vi "Serial Verify.vi"(6 "Function Choose":T3(ring), 8 "error in (no error)":errorcluster, 9 "Config Parameters":T1={"HEX_Max"="1A", "HEX_Min"="", "Read?"=FALSE, "write buffer"="", "Wait Time(ms)"=0}, 10 "Serial Config":T2={"baud rate (9600)"=9600, "stop bits (10: 1 bit)"=10, "flow control (0:none)"=0, "data bits (8)"=8, "parity (0:none)"=enum."None"} {"data bits (8)" min=5 max=8 step=1; "flow control (0:none)" items=["None", "XON/XOFF", "RTS/CTS", "XON/XOFF & RTS/CTS", "DTR/DSR", "XON/XOFF & DTR/DSR"]; "stop bits (10: 1 bit)" items=["1.0"=10, "1.5"=15, "2.0"=20]}, 11 "VISA resource name":refnum<visa-resource-name>) -> (0 "error out":errorcluster, 2 "Result":string, 3 "VISA resource name out":refnum<visa-resource-name>)   [LabVIEW 2020]
uses:
  6da304eb-4ed6-4a05-99e3-1c15b644af6c.vi
  a31ce7cd-64d5-4b98-9705-88e585e787fb.vi
  <vilib>/Instr/_visa.llb/VISA Configure Serial Port (Instr).vi
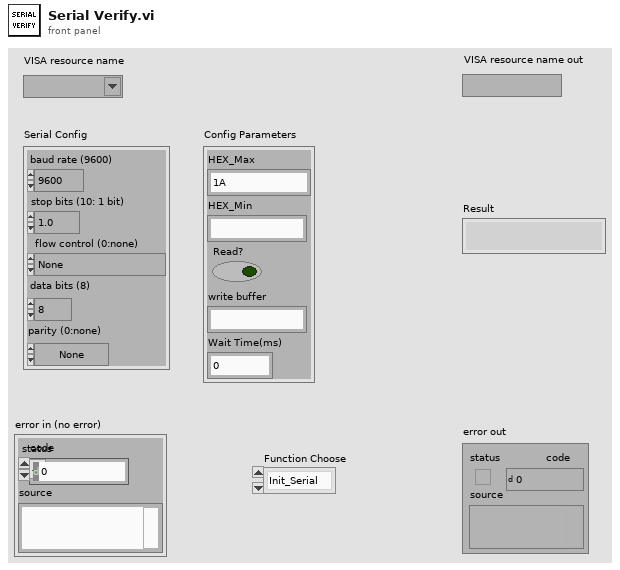
[diagram p1: front panel]
types:
  T1 = cluster{"HEX_Max":string, "HEX_Min":string, "Read?":bool, "write buffer":string, "Wait Time(ms)":u32}
  T2 = cluster{"baud rate (9600)":u32, "stop bits (10: 1 bit)":u16, "flow control (0:none)":u16, "data bits (8)":u16, "parity (0:none)":enum16{"None", "Odd", "Even", "Mark", "Space"}}
  T3 = enum16{"Init_Serial", "Write&Read", "Check_Value", "Close_Serial"}
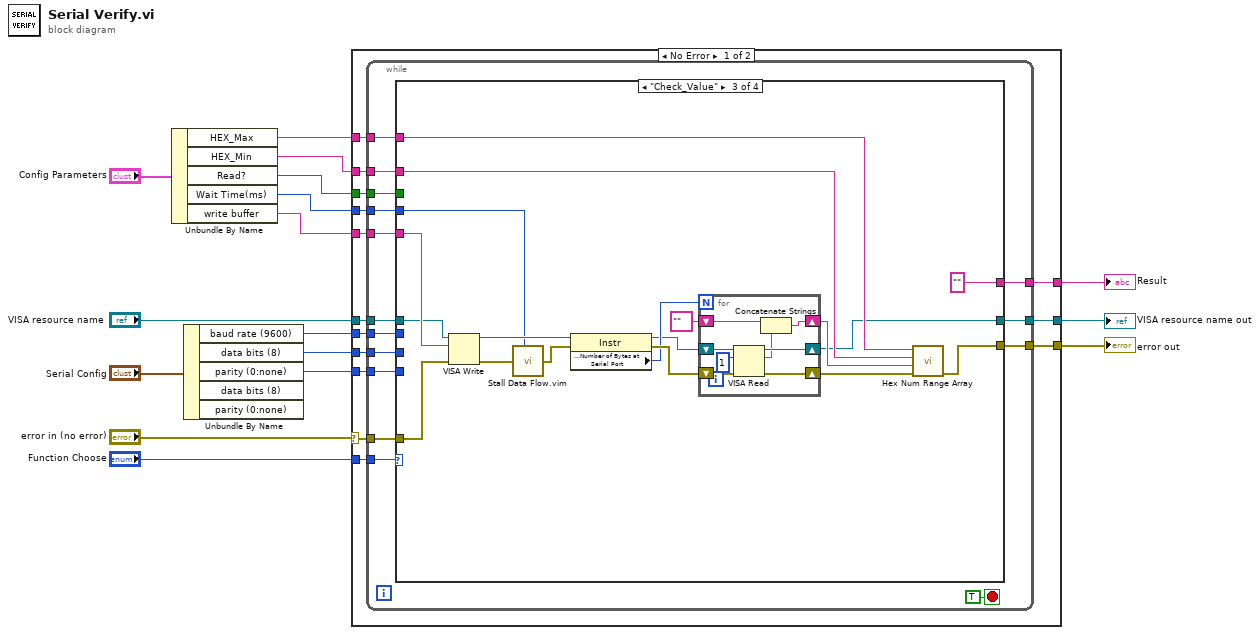
[diagram p0: block diagram]
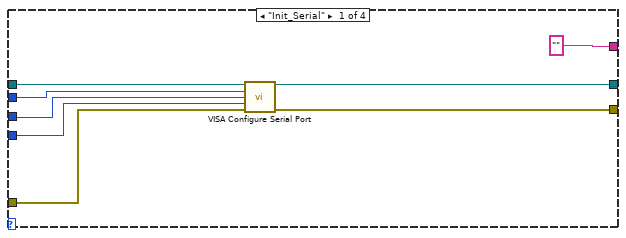
[diagram p2: hidden frame]
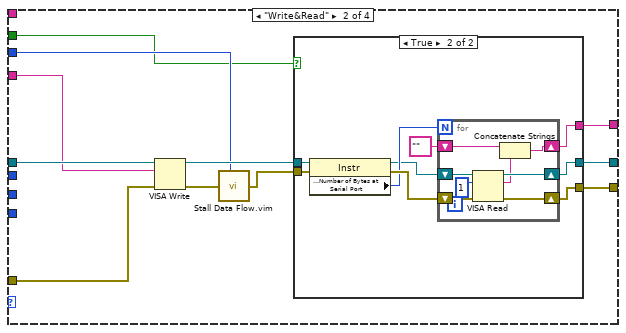
[diagram p3: hidden frame]
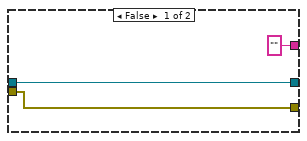
[diagram p4: hidden frame]
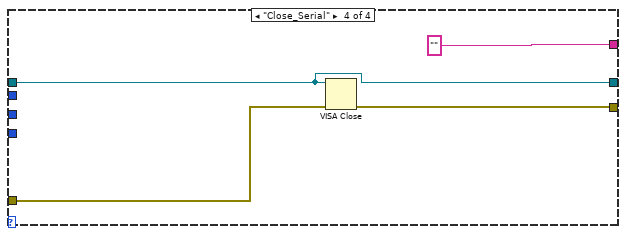
[diagram p5: hidden frame]
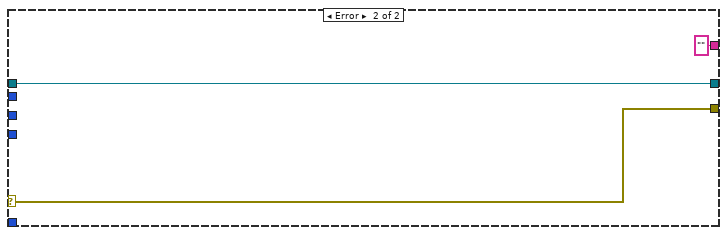
[diagram p6: hidden frame]
diagram:
  n1 = Unbundle By Name("Config Parameters") -> ("HEX_Max"=w5:string, "HEX_Min"=w4:string, "Read?"=w3:bool, "Wait Time(ms)"=w2:u32, "write buffer"=w1:string)
  n2 = Unbundle By Name("Serial Config") -> ("baud rate (9600)"=w12:u32, "data bits (8)"=w11:u16, "parity (0:none)"=w10:enum16{"None", "Odd", "Even", "Mark", "Space"})  [unwired: 2 out]
  n3 = case shown="No Error" "error in (no error)" {
    selector: "error in (no error)" -> [w25 w115]
    tunnel: "Function Choose" -> [w30 _]
    tunnel: "VISA resource name" -> [w29 w116]
    tunnel: w12 -> [w28 _]
    tunnel: w11 -> [w27 _]
    tunnel: w10 -> [w26 _]
    tunnel: [w24 w115] -> w9
    tunnel: [w23 w116] -> w8
    tunnel: w2 -> [w22 _]
    tunnel: w1 -> [w21 _]
    tunnel: [w20 ""] -> w7
    tunnel: w3 -> [w19 _]
    tunnel: w5 -> [w18 _]
    tunnel: w4 -> [w17 _]
    frame No Error {
      n4 = while {
        tunnel: w30 -> [w37]
        tunnel: w29 -> [w44]
        tunnel: w28 -> [w43]
        tunnel: w27 -> [w42]
        tunnel: w26 -> [w41]
        tunnel: w25 -> [w40]
        tunnel: [w39] -> w24
        tunnel: [w38] -> w23
        tunnel: w22 -> [w36]
        tunnel: w21 -> [w35]
        tunnel: [w34] -> w20
        tunnel: w19 -> [w33]
        tunnel: w18 -> [w32]
        tunnel: w17 -> [w31]
        stop <- TRUE stop-if-true
        n5 = case shown="\"Check_Value\"" w37 {
          tunnel: w44 -> [w53 w64 w93 w112]
          tunnel: w43 -> [w52 _ _ _]
          tunnel: w42 -> [w51 _ _ _]
          tunnel: w41 -> [w50 _ _ _]
          tunnel: w40 -> [w49 w63 w95 w114]
          tunnel: [w48 w54 w87 w113] -> w39
          tunnel: [w47 w55 w86 w112] -> w38
          tunnel: w36 -> [_ w59 w92 _]
          tunnel: w35 -> [_ w58 w94 _]
          tunnel: ["" w57 "" ""] -> w34
          tunnel: w33 -> [_ w56 _ _]
          tunnel: w32 -> [_ _ w90 _]
          tunnel: w31 -> [_ _ w89 _]
          frame "Init_Serial" {
            n6 = call-poly "VISA Configure Serial Port"("VISA resource name"=w53, "baud rate (9600)"=w52, "data bits (8)"=w51, "parity (0:none)"=w50, "error in (no error)"=w49) -> ("VISA resource name out"=w47:refnum<visa-resource-name>, "error out"=w48:errorcluster)  [unwired: 9 in]
          }
          frame "Write&Read" {
            n7 = VISA Write(VISA resource name=w64, write buffer=w58, error in (no error)=w63) -> (VISA resource name out=w60:refnum<visa-resource-name>, error out=w62:errorcluster)  [unwired: 1 out]
            n8 = call "Stall Data Flow.vim"("value in"=w62, "milliseconds to wait"=w59) -> ("value out"=w61:errorcluster)  [unwired: 1 out]
            n9 = case shown="True" w56 {
              tunnel: w61 -> [w66 w72]
              tunnel: w60 -> [w67 w71]
              tunnel: ["" w70] -> w57
              tunnel: [w67 w69] -> w55
              tunnel: [w66 w68] -> w54
              frame False {
              }
              frame True {
                n10 = property class="Instr"(reference=w71, error in=w72) -> (reference out=w74:refnum<visa-resource-name>, error out=w76:errorcluster, "Serial Settings:Number of Bytes at Serial Port"=w75:u32)
                n11 = for {
                  N: w75 -> [_]
                  shift-right: [w80] -> w69
                  shift-left: w74 -> [w82]
                  shift-right: [w77] -> w70
                  shift-left: "" -> [w78]
                  shift-right: [w81] -> w68
                  shift-left: w76 -> [w83]
                  n12 = VISA Read(VISA resource name=w82, byte count=u32 1, error in (no error)=w83) -> (VISA resource name out=w80:refnum<visa-resource-name>, read buffer=w79:string, error out=w81:errorcluster)  [unwired: 1 out]
                  n13 = Concatenate Strings(w78, w79) -> (w77:string)
                }
              }
            }
          }
          frame "Check_Value" {
            n14 = VISA Write(VISA resource name=w93, write buffer=w94, error in (no error)=w95) -> (VISA resource name out=w100:refnum<visa-resource-name>, error out=w102:errorcluster)  [unwired: 1 out]
            n15 = call "Stall Data Flow.vim"("value in"=w102, "milliseconds to wait"=w92) -> ("value out"=w101:errorcluster)  [unwired: 1 out]
            n16 = property class="Instr"(reference=w100, error in=w101) -> (reference out=w97:refnum<visa-resource-name>, error out=w99:errorcluster, "Serial Settings:Number of Bytes at Serial Port"=w98:u32)
            n17 = for {
              N: w98 -> [_]
              shift-right: [w106] -> w86
              shift-left: w97 -> [w108]
              shift-right: [w103] -> w88
              shift-left: "" -> [w104]
              shift-right: [w107] -> w91
              shift-left: w99 -> [w109]
              n18 = VISA Read(VISA resource name=w108, byte count=u32 1, error in (no error)=w109) -> (VISA resource name out=w106:refnum<visa-resource-name>, read buffer=w105:string, error out=w107:errorcluster)  [unwired: 1 out]
              n19 = Concatenate Strings(w104, w105) -> (w103:string)
            }
            n20 = call "Hex Num Range Array.vi"("error in (no error)"=w91, "Check String"=w88, "HEX_Min"=w89, "HEX_Max"=w90) -> ("error out"=w87:errorcluster)  [unwired: 5 in, 2 out]
          }
          frame "Close_Serial" {
            n21 = VISA Close(VISA resource name=w112, error in (no error)=w114) -> (error out=w113:errorcluster)
          }
        }
      }
    }
    frame Error {
    }
  }
  "Result" <- w7
  "error out" <- w9
  "VISA resource name out" <- w8
